vi "CalculateDelay_From_Fi_korr.vi"(8 "input valid":bool=TRUE, 10 "fi_korr":fxp<+/-,32,4>, 11 "Data in":fxp<+/-,16,14>[](array[numeric])=[0.0, 0.0, 0.0, 0.0]) -> (0 "output valid":bool, 3 "Data out":fxp<+/-,16,14>[](array[numeric]))   [LabVIEW 2013]
doc: "Calculates various combinations on I_in, Q_in and cos(fi) and sin(fi) to be used later to delay the output signal"
uses:
  <vilib>/rvi/FXPMathLib/FxpSinAndCos/subVIs/nifxpmath_SinAndCos_SimConfig.ctl
  <vilib>/rvi/FXPMathLib/FxpSinAndCos/simVIs/DllFxpSinAndCosTemp_sub.vi
  <vilib>/rvi/FXPMathLib/FxpSinAndCos/XNode/nifxpmath_SinAndCos.xnode
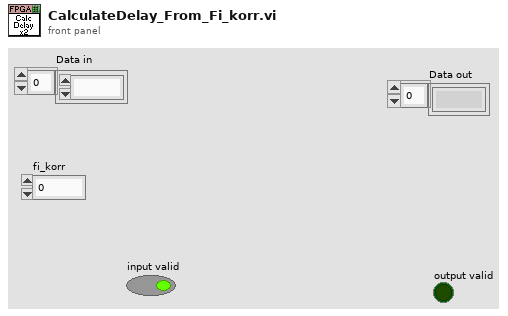
[diagram p1: front panel]
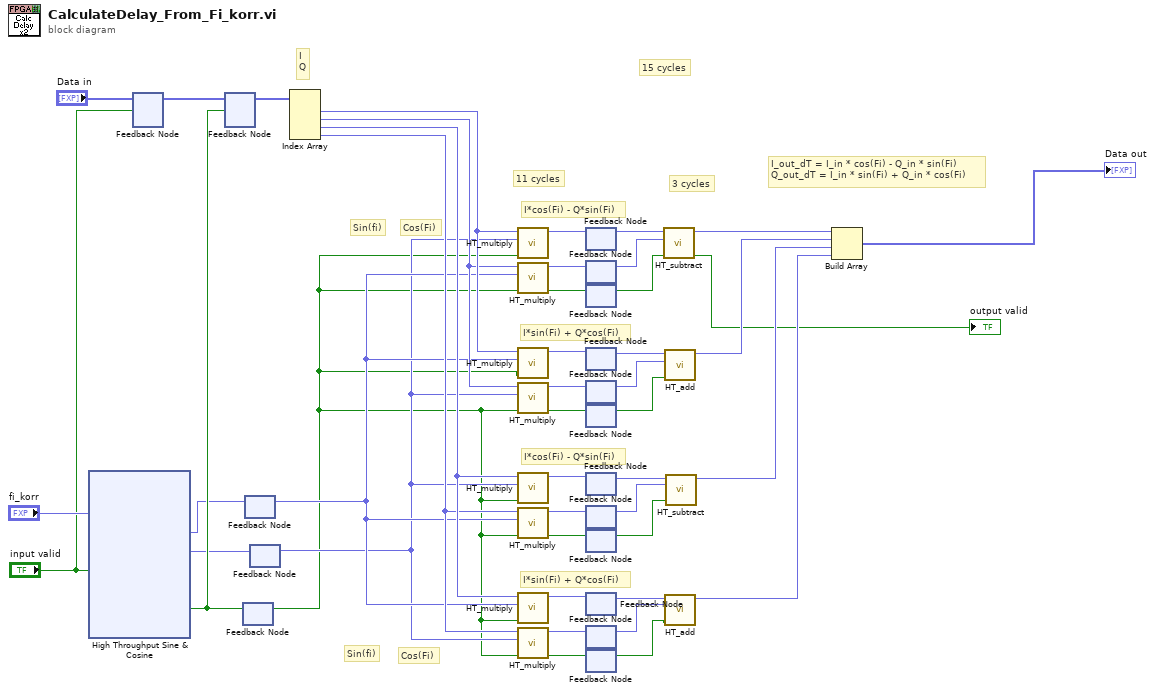
[diagram p0: block diagram]
diagram:
  # "I*sin(Fi) + Q*cos(Fi)"
  # "I*cos(Fi) - Q*sin(Fi)"
  # "Cos(Fi)"
  # "Sin(fi)"
  # "Cos(Fi)"
  # "Sin(fi)"
  # "I_out_dT = I_in * cos(Fi) - Q_in * sin(Fi)\nQ_out_dT = I_in * sin(Fi) + Q_in * cos(Fi)"
  # "3 cycles"
  # "11 cycles"
  # "15 cycles"
  # "I*sin(Fi) + Q*cos(Fi)"
  # "I\nQ"
  # "I*cos(Fi) - Q*sin(Fi)"
  n1 = xnode "High Throughput Sine & Cosine"("x (pi)"="fi_korr", "input valid"="input valid") -> ("sin(x)"=w5:fxp<+/-,16,2>, "cos(x)"=w4:fxp<+/-,16,2>, "output valid"=w6:bool)  [unwired: 1 in, 1 out]
  n2 = feedback #1() -> (w1:fxp<+/-,16,14>[])  [unwired: 1 in]
  n3 = feedback-in #1("Data in", "input valid") -> ()
  n4 = feedback #2() -> (w3:fxp<+/-,16,14>[])  [unwired: 1 in]
  n5 = feedback-in #2(w1, w6) -> ()
  n6 = feedback #3() -> (w8:bool)  [unwired: 1 in]
  n7 = feedback-in #3(w6) -> ()
  n8 = feedback #4() -> (w11:fxp<+/-,16,2>)  [unwired: 1 in]
  n9 = feedback-in #4(w5) -> ()
  n10 = feedback #5() -> (w9:fxp<+/-,16,2>)  [unwired: 1 in]
  n11 = feedback-in #5(w4) -> ()
  n12 = Index Array(array=w3) -> (element #1=w39:fxp<+/-,16,14>, element #2=w38:fxp<+/-,16,14>, element #3=w13:fxp<+/-,16,14>, element #4=w12:fxp<+/-,16,14>)  [unwired: 4 in]
  n13 = call "HT_multiply.vi"("input valid"=w8, "y"=w9, "x"=w39) -> ("x*y"=w45:fxp<+/-,16,14>)  [unwired: 7 in, 1 out]
  n14 = call "HT_multiply.vi"("input valid"=w8, "y"=w11, "x"=w38) -> ("output valid"=w43:bool, "x*y"=w44:fxp<+/-,16,14>)  [unwired: 7 in]
  n15 = call "HT_multiply.vi"("input valid"=w8, "y"=w11, "x"=w39) -> ("x*y"=w40:fxp<+/-,16,14>)  [unwired: 7 in, 1 out]
  n16 = call "HT_multiply.vi"("input valid"=w8, "y"=w9, "x"=w38) -> ("output valid"=w42:bool, "x*y"=w41:fxp<+/-,16,14>)  [unwired: 7 in]
  n17 = call "HT_multiply.vi"("input valid"=w8, "y"=w9, "x"=w13) -> ("x*y"=w31:fxp<+/-,16,14>)  [unwired: 7 in, 1 out]
  n18 = call "HT_multiply.vi"("input valid"=w8, "y"=w11, "x"=w12) -> ("output valid"=w33:bool, "x*y"=w32:fxp<+/-,16,14>)  [unwired: 7 in]
  n19 = call "HT_multiply.vi"("input valid"=w8, "y"=w11, "x"=w13) -> ("x*y"=w36:fxp<+/-,16,14>)  [unwired: 7 in, 1 out]
  n20 = call "HT_multiply.vi"("input valid"=w8, "y"=w9, "x"=w12) -> ("output valid"=w34:bool, "x*y"=w35:fxp<+/-,16,14>)  [unwired: 7 in]
  n21 = feedback #6() -> (w18:fxp<+/-,16,14>)  [unwired: 1 in]
  n22 = feedback-in #6(w45) -> ()
  n23 = feedback #7() -> (w14:fxp<+/-,16,14>)  [unwired: 1 in]
  n24 = feedback-in #7(w44) -> ()
  n25 = feedback #8() -> (w15:bool)  [unwired: 1 in]
  n26 = feedback-in #8(w43) -> ()
  n27 = feedback #9() -> (w20:fxp<+/-,16,14>)  [unwired: 1 in]
  n28 = feedback-in #9(w40) -> ()
  n29 = feedback #10() -> (w21:fxp<+/-,16,14>)  [unwired: 1 in]
  n30 = feedback-in #10(w41) -> ()
  n31 = feedback #11() -> (w22:bool)  [unwired: 1 in]
  n32 = feedback-in #11(w42) -> ()
  n33 = feedback #12() -> (w25:fxp<+/-,16,14>)  [unwired: 1 in]
  n34 = feedback-in #12(w31) -> ()
  n35 = feedback #13() -> (w24:fxp<+/-,16,14>)  [unwired: 1 in]
  n36 = feedback-in #13(w32) -> ()
  n37 = feedback #14() -> (w23:bool)  [unwired: 1 in]
  n38 = feedback-in #14(w33) -> ()
  n39 = feedback #15() -> (w30:fxp<+/-,16,14>)  [unwired: 1 in]
  n40 = feedback-in #15(w36) -> ()
  n41 = feedback #16() -> (w29:fxp<+/-,16,14>)  [unwired: 1 in]
  n42 = feedback-in #16(w35) -> ()
  n43 = feedback #17() -> (w28:bool)  [unwired: 1 in]
  n44 = feedback-in #17(w34) -> ()
  n45 = call "HT_subtract.vi"("input valid"=w15, "y"=w14, "x"=w18) -> ("output valid"=→"output valid":bool, "x+y"=w17:fxp<+/-,16,14>)  [unwired: 7 in]
  n46 = call "HT_add.vi"("input valid"=w22, "y"=w21, "x"=w20) -> ("x+y"=w19:fxp<+/-,16,14>)  [unwired: 7 in, 1 out]
  n47 = call "HT_add.vi"("input valid"=w28, "y"=w29, "x"=w30) -> ("x+y"=w27:fxp<+/-,16,14>)  [unwired: 7 in, 1 out]
  n48 = call "HT_subtract.vi"("input valid"=w23, "y"=w24, "x"=w25) -> ("x+y"=w26:fxp<+/-,16,14>)  [unwired: 7 in, 1 out]
  n49 = Build Array(w17, w19, w26, w27) -> (→"Data out":fxp<+/-,16,14>[])
